vi "testRotHexaPos.vi"(8 "error in (no error)":errorcluster) -> (0 "error out":errorcluster)   [LabVIEW 2016]
doc: "Test the rotation of hexapod position (degree of freedom, DOF) with the non-zero camera rotation angle."
uses:
  CamRot/CamRot.lvclass
  StrictDef/DofGroup.ctl
  <vilib>/addons/_JKI Toolkits/Caraya/classes/Test/Test.lvclass
  <vilib>/addons/_JKI Toolkits/Caraya/classes/Assert/Assert.lvclass
panel:
  in  "CamRot.lvclass":refnum<class "CamRot.lvclass">
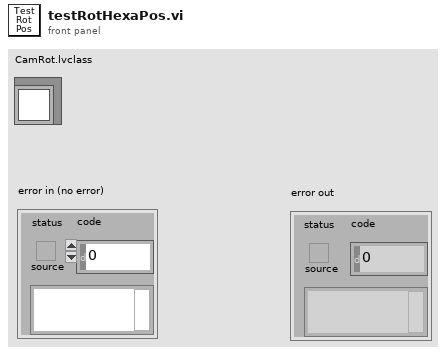
[diagram p1: front panel]
types:
  T1 = typedef "DofGroup.ctl" = enum16{"M2 Hex Pos", "Cam Hex Pos", "M1M3 Bend", "M2 Bend"}
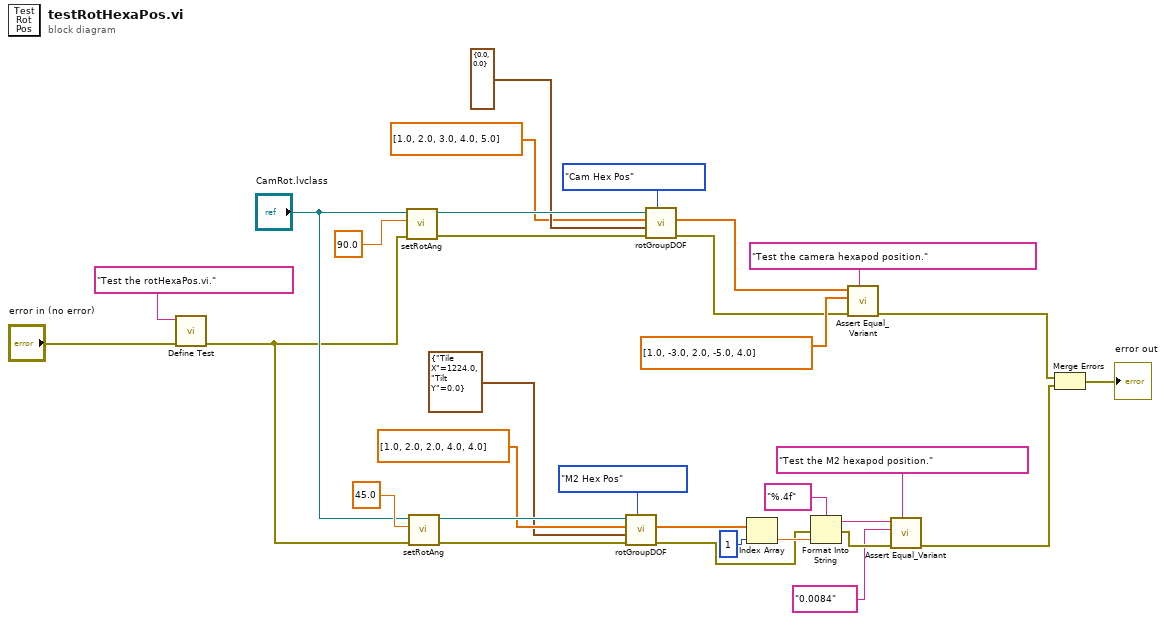
[diagram p0: block diagram]
diagram:
  n1 = call <vilib>:"Define Test.vi"("error in (no error)"="error in (no error)", "Label (VI Title)"="Test the rotHexaPos.vi.") -> ("error out"=w26:errorcluster)  [unwired: 9 in]
  n2 = call "setRotAng.vi"("error in (no error)"=w26, "Rotation Angle in Deg"=90.0, "CamRot in"="CamRot.lvclass") -> ("error out"=w10:errorcluster, "CamRot out"=w14:refnum<class "CamRot.lvclass">)  [unwired: 7 in]
  n3 = call "setRotAng.vi"("error in (no error)"=w26, "Rotation Angle in Deg"=45.0, "CamRot in"="CamRot.lvclass") -> ("error out"=w3:errorcluster, "CamRot out"=w7:refnum<class "CamRot.lvclass">)  [unwired: 7 in]
  n4 = call "rotGroupDOF.vi"("DOF Group"=DofGroup."M2 Hex Pos", "error in (no error)"=w3, "Tilt Angle (arcsec)"=cluster{"Tile X":dbl, "Tilt Y":dbl} {"Tile X"=1224.0, "Tilt Y"=0.0}, "State in DOF"=dbl[] [1.0, 2.0, 2.0, 4.0, 4.0] ("Hexapod DOF"), "CamRot in"=w7) -> ("error out"=w2:errorcluster, "Rotated State in DOF"=w1:dbl[])  [unwired: 4 in, 1 out]
  n5 = call "rotGroupDOF.vi"("DOF Group"=DofGroup."Cam Hex Pos", "error in (no error)"=w10, "Tilt Angle (arcsec)"=cluster{"Tile X":dbl, "Tilt Y":dbl} {"Tile X"=0.0, "Tilt Y"=0.0}, "State in DOF"=dbl[] [1.0, 2.0, 3.0, 4.0, 5.0] ("Hexapod DOF"), "CamRot in"=w14) -> ("error out"=w8:errorcluster, "Rotated State in DOF"=w9:dbl[])  [unwired: 4 in, 1 out]
  n6 = Index Array(array=w1, index=1) -> (element=w21:dbl)
  n7 = Format Into String(format string="%.4f" ("initial string"), error in=w2, w21) -> (resulting string=w19:string, error out=w17:errorcluster)  [unwired: 1 in]
  n8 = call <vilib>:"Assert Equal_Variant.vi"("Label"="Test the camera hexapod position.", "error in (no error)"=w8, "Y"=dbl[] [1.0, -3.0, 2.0, -5.0, 4.0] ("Hexapod DOF"), "X"=w9) -> ("error out"=w23:errorcluster)  [unwired: 7 in]
  n9 = call <vilib>:"Assert Equal_Variant.vi"("Label"="Test the M2 hexapod position.", "error in (no error)"=w17, "Y"="0.0084" ("Label"), "X"=w19) -> ("error out"=w16:errorcluster)  [unwired: 7 in]
  n10 = Merge Errors(w23, w16) -> (→"error out":errorcluster)
